vi "Host Approach RetractionA1copy-Aidan.vi"() -> ()   [LabVIEW 2012]
uses:
  <vilib>/Utility/file.llb/Write To Spreadsheet File (I64).vi
  <vilib>/FPGAPlugInAG/PCI-7831R/niLvFpga_Open_PCI-7831R.vi
  <vilib>/rvi/interface/common/dynamic/niFpgaDynamicAddResources.vi
  <vilib>/FPGAPlugInAG/Dynamic/niLvFpga_Run_Dynamic.vi
  <vilib>/Utility/error.llb/Error Cluster From Error Code.vi
  <vilib>/rvi/errors/niLvFpgaAdjustHostInterfaceError.vi
  <vilib>/FPGAPlugInAG/Dynamic/niLvFpga_Close_Dynamic.vi
  <vilib>/rvi/interface/nirviOpenFPGA/nirviOpenFPGA.xnode
  SB130-XPS/Documents/FPGA-project-apporach-retraction/FPGA Bitfiles/Apporach-Retract_FPGATarget2_FPGATargetApproa_sPWXUlF8ZuM.lvbitx
  Downloads/FPGA Target Approach RetractionA2copyAidanV2.vi
  <vilib>/rvi/interface/nirviMethod/nirviMethod.xnode
  <vilib>/rvi/interface/nirviReadWriteControl/nirviReadWriteControl.xnode
  <vilib>/rvi/interface/nirviCloseFPGA/nirviCloseFPGA.xnode
  <vilib>/rvi/interface/Simulation/niFpgaSimulationCallBeginRW.vi
  <vilib>/rvi/errors/niLvFpgaMergeErrorWithErrorCode.vi
  <vilib>/FPGAPlugInAG/Dynamic/niLvFpga_StartFifo_Dynamic.vi
  <vilib>/FPGAPlugInAG/Dynamic/niLvFpga_StopFifo_Dynamic.vi
  <vilib>/FPGAPlugInAG/Dynamic/niLvFpga_ReadFifo_Dynamic.vi
  NiFpgaLv.dll
panel:
  out "Acoustic Signal":u32[](graph)
  out "Acoustic Signal Data":i16[](array[numeric])
  in  "PANIC Retract\n\nApproach must be\n off before using":bool
  in  "File Name":string
  in  "Base Path":path
  in  "Colllect Data?":bool
  out "Counter Indicator Data":u16[](array[numeric])
  out "Total Error Data":u16[](array[numeric])
  out "Error Data":i16[](array[numeric])
  out "HV/10 Data":i16[](array[numeric])
  out "Tuning Fork \nSignal data":u16[](array[numeric])
  out "Counter Indicator":u32[](graph)
  out "Total Error":u16[](graph)
  out "Error":u16[](graph)
  out "Tuning Fork Signal":u16[](graph)
  out "HV/10":u16[](graph)
  out "Data 2":u64[](array[numeric])
  out "Data 1":u64[](array[numeric])
  in  "Intergral Constant":i32
  in  "Porportional Constant":i32
  in  "Feedback":bool
  in  "Approach Minimum":i32=20000
  in  "Approach Setpoint":i32=23000
  in  "Fast Approach Offset":i32=29000
  in  "TF in Air":i32=36000
  out "Fine A bits/us":dbl=5.463300000000001e-06
  out "Fine R bits/us":dbl=5.463300000000001e-06
  in  "Fine Approach (nm/s)":dbl=5.0
  in  "Fine Retraction (nm/s)":dbl=5.0
  out "Boolean 2":bool
  in  "DAQ Rate":i32=8000
  in  "Number of Elements":i32=100
  out "Fast A nm/s indicator":dbl=200.0
  out "Fast A bits/us":dbl=0.00021853200000000001
  out "Fast R nm/s indicator":dbl=200.0
  out "Fast R bits/us":dbl=0.00021853200000000001
  in  "Fast Approach (nm/s)":dbl=200.0
  in  "Fast Retraction (nm/s)":dbl=200.0
  in  "Automated Approach Start":bool
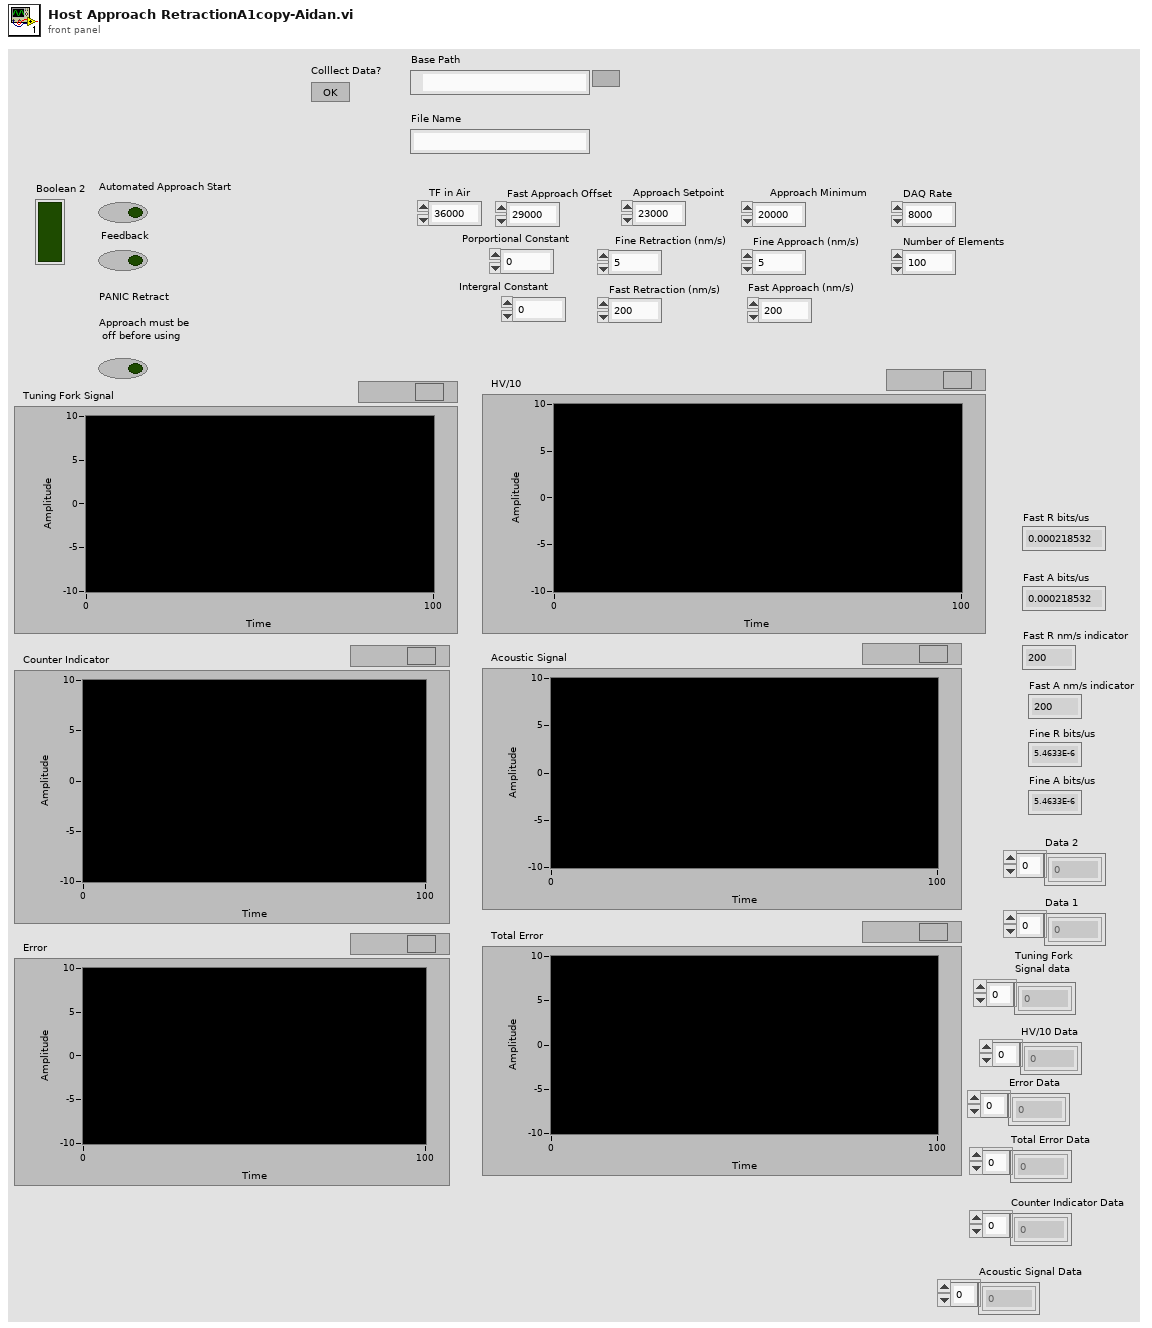
[diagram p1: front panel]
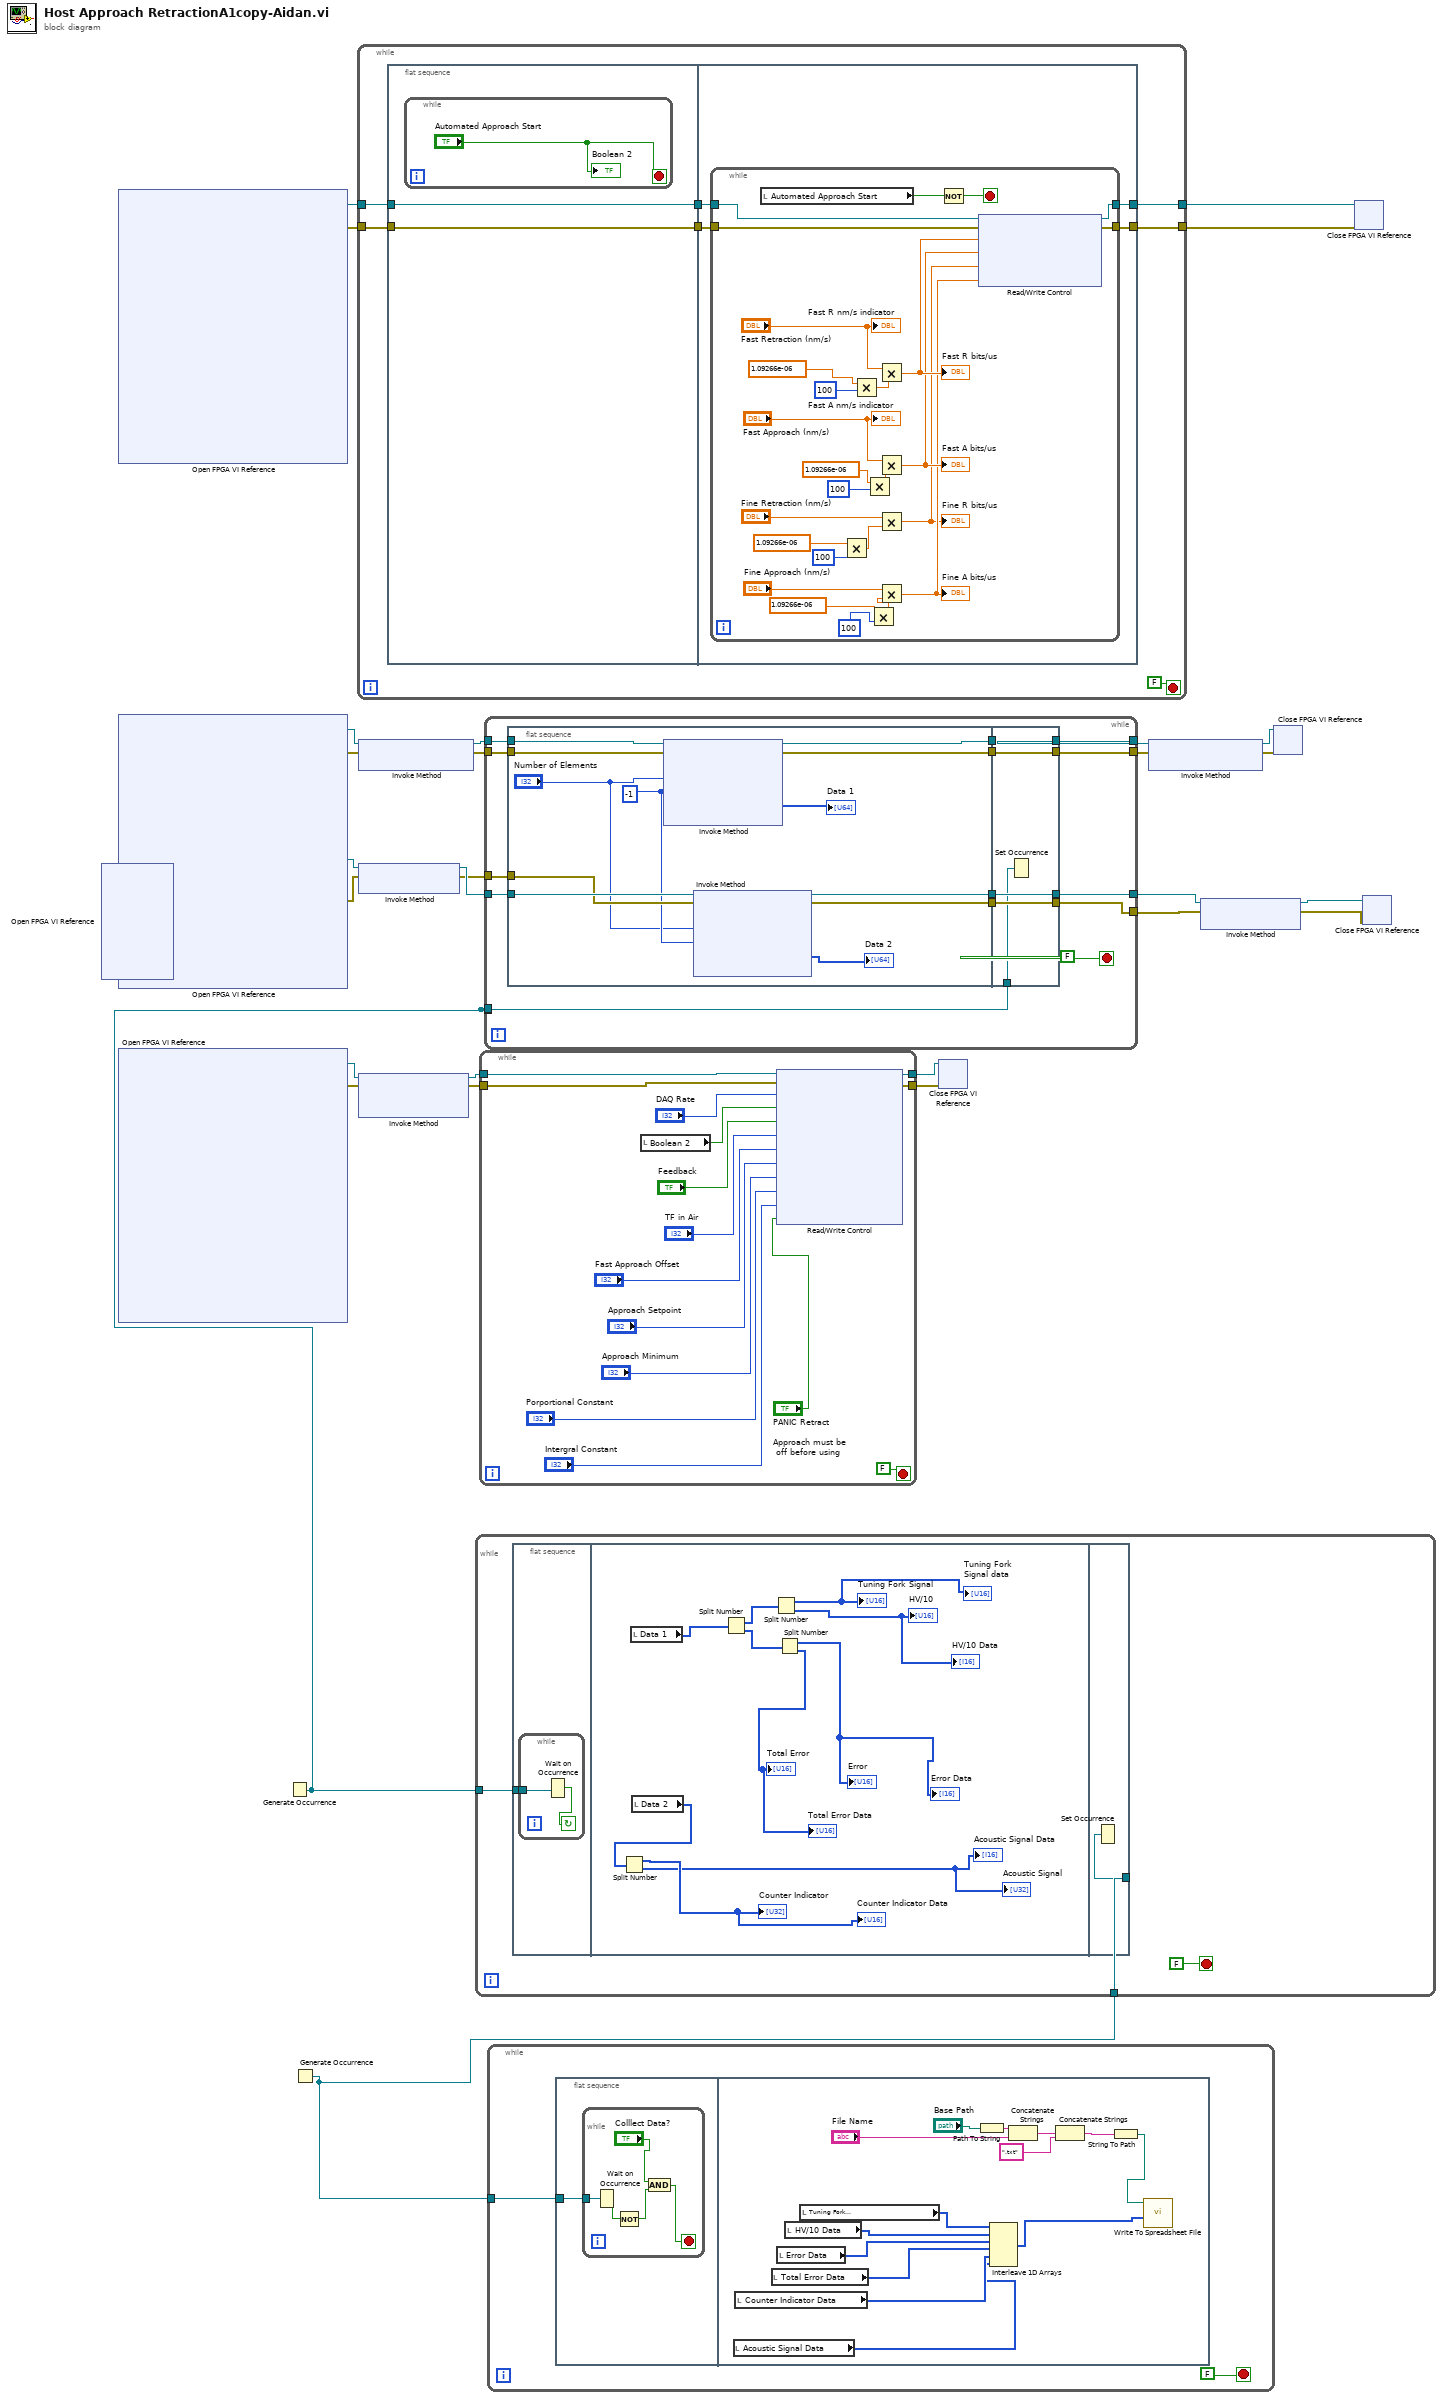
[diagram p0: block diagram]
diagram:
  n1 = xnode "Open FPGA VI Reference"() -> ("FPGA VI Reference Out"=w11:refnum<k20>, "error out"=w10:errorcluster)  [unwired: 2 in]
  n2 = xnode ("Open FPGA VI Reference")() -> ("FPGA VI Reference Out"=w23:refnum<k20>, "error out"=w22:errorcluster)  [unwired: 2 in]
  n3 = xnode "Open FPGA VI Reference"() -> ("FPGA VI Reference Out"=w9:refnum<k20>, "error out"=w19:errorcluster)  [unwired: 2 in]
  n4 = xnode "Open FPGA VI Reference"() -> ("FPGA VI Reference Out"=w24:refnum<k20>, "error out"=w12:errorcluster)  [unwired: 2 in]
  n5 = Generate Occurrence() -> (w2:refnum<k4>)
  n6 = Generate Occurrence() -> (w1:refnum<k4>)
  n7 = while {
    tunnel: w23 -> [w34]
    tunnel: w22 -> [w33]
    tunnel: [w30] -> w21
    tunnel: [w29] -> w20
    stop <- FALSE stop-if-true
    n8 = flat-sequence {
      tunnel: w34 -> [w37]
      tunnel: w33 -> [w36]
      tunnel: [w37] -> w32
      tunnel: [w36] -> w31
      tunnel: w32 -> [w42]
      tunnel: w31 -> [w41]
      tunnel: [w40] -> w30
      tunnel: [w39] -> w29
      frame #0 {
        n9 = while {
          stop <- "Automated Approach Start" stop-if-true
          "Boolean 2" <- "Automated Approach Start"
        }
      }
      frame #1 {
        n10 = while {
          tunnel: w42 -> [w62]
          tunnel: w41 -> [w61]
          tunnel: [w64] -> w40
          tunnel: [w63] -> w39
          stop <- w68 stop-if-true
          n11 = local read "Automated Approach Start"() -> (w67:bool)
          n12 = Multiply(x=1.09266e-06, y=100) -> (x*y=w47:dbl)
          n13 = Multiply(x=1.09266e-06, y=100) -> (x*y=w53:dbl)
          n14 = Multiply(x=1.09266e-06, y=100) -> (x*y=w50:dbl)
          n15 = Multiply(x=1.09266e-06, y=100) -> (x*y=w43:dbl)
          n16 = Multiply(x="Fast Retraction (nm/s)", y=w53) -> (x*y=w60:dbl)
          "Fast R bits/us" <- w60
          n17 = Multiply(x="Fast Approach (nm/s)", y=w50) -> (x*y=w59:dbl)
          "Fast A bits/us" <- w59
          n18 = Multiply(x="Fine Retraction (nm/s)", y=w47) -> (x*y=w55:dbl)
          "Fine R bits/us" <- w55
          n19 = Multiply(x="Fine Approach (nm/s)", y=w43) -> (x*y=w56:dbl)
          "Fine A bits/us" <- w56
          n20 = Not(x=w67) -> (.not. x?=w68:bool)
          n21 = xnode "Read/Write Control"("FPGA VI Reference In"=w62, "error in"=w61, "Fast Retraction Speed"=w60, "Fast Approach Speed"=w59, "Fine Retraction Speed"=w55, "Fine Approach Speed"=w56) -> ("FPGA VI Reference Out"=w64:refnum<k20>, "error out"=w63:errorcluster)
          "Fast R nm/s indicator" <- "Fast Retraction (nm/s)"
          "Fast A nm/s indicator" <- "Fast Approach (nm/s)"
        }
      }
    }
  }
  n22 = xnode "Invoke Method"("FPGA VI Reference In"=w9, "error in"=w19) -> ("FPGA VI Reference Out"=w18:refnum<k20>, "error out"=w17:errorcluster)
  n23 = xnode "Invoke Method"("FPGA VI Reference In"=w11, "error in"=w10) -> ("FPGA VI Reference Out"=w8:refnum<k20>, "error out"=w7:errorcluster)
  n24 = xnode "Invoke Method"("FPGA VI Reference In"=w24, "error in"=w12) -> ("FPGA VI Reference Out"=w26:refnum<k20>, "error out"=w25:errorcluster)  [unwired: 1 in]
  n25 = while {
    tunnel: w2 -> [w70]
    tunnel: w1 -> [w69]
    stop <- FALSE stop-if-true
    n26 = flat-sequence {
      tunnel: w70 -> [w72]
      tunnel: w69 -> [w85]
      frame #0 {
        n27 = while {
          tunnel: w72 -> [w74]
          stop <- w73 continue-if-true
          n28 = Wait on Occurrence(2:w74) -> (0:w73:bool)  [unwired: 2 in]
        }
      }
      frame #1 {
        n29 = local read "Data 1"() -> (w84:u64[])
        n30 = local read "Data 2"() -> (w77:u64[])
        n31 = Split Number(x=w77) -> (hi(x)=→"Counter Indicator" →"Counter Indicator Data":u32[], lo(x)=→"Acoustic Signal Data" →"Acoustic Signal":u32[])
        n32 = Split Number(x=w84) -> (hi(x)=w83:u32[], lo(x)=w82:u32[])
        n33 = Split Number(x=w83) -> (hi(x)=→"Tuning Fork Signal" →"Tuning Fork \nSignal data":u16[], lo(x)=→"HV/10" →"HV/10 Data":u16[])
        n34 = Split Number(x=w82) -> (hi(x)=→"Error" →"Error Data":u16[], lo(x)=→"Total Error" →"Total Error Data":u16[])
      }
      frame #2 {
        n35 = Set Occurrence(w85) -> ()
      }
    }
  }
  n36 = while {
    tunnel: w26 -> [w99]
    tunnel: w25 -> [w98]
    tunnel: [w97] -> w28
    tunnel: [w96] -> w27
    stop <- FALSE stop-if-true
    n37 = local read "Boolean 2"() -> (w94:bool)
    n38 = xnode "Read/Write Control"("FPGA VI Reference In"=w99, "error in"=w98, "Data Acquisition Rate"="DAQ Rate", "Approach"=w94, "Feedback?"="Feedback", "TF in Air"="TF in Air", "Fast Approach Offset"="Fast Approach Offset", "Approach Setpoint"="Approach Setpoint", "Approach Minimum"="Approach Minimum", "Porportional Constant"="Porportional Constant", "Integral Constant"="Intergral Constant", "PANIC Retract"="PANIC Retract\n\nApproach must be\n off before using") -> ("FPGA VI Reference Out"=w97:refnum<k20>, "error out"=w96:errorcluster)
  }
  n39 = while {
    tunnel: w18 -> [w114]
    tunnel: w17 -> [w113]
    tunnel: [w112] -> w16
    tunnel: [w111] -> w15
    tunnel: w8 -> [w109]
    tunnel: w7 -> [w108]
    tunnel: [w107] -> w6
    tunnel: [w106] -> w5
    tunnel: w2 -> [_]
    tunnel: w2 -> [w101]
    stop <- FALSE stop-if-true
    n40 = flat-sequence {
      tunnel: w114 -> [w126]
      tunnel: w113 -> [w125]
      tunnel: w109 -> [w122]
      tunnel: w108 -> [w121]
      tunnel: [w124] -> w105
      tunnel: [w123] -> w104
      tunnel: [w118] -> w103
      tunnel: [w117] -> w102
      tunnel: [w128] -> w106
      tunnel: [w129] -> w107
      tunnel: [w130] -> w111
      tunnel: [w131] -> w112
      tunnel: w105 -> [w131]
      tunnel: w104 -> [w130]
      tunnel: w103 -> [w129]
      tunnel: w102 -> [w128]
      tunnel: w101 -> [w127]
      frame #0 {
        w120 = -1
        n41 = xnode "Invoke Method"("FPGA VI Reference In"=w126, "error in"=w125, "Number of Elements"="Number of Elements", "Timeout (ms)"=w120) -> ("FPGA VI Reference Out"=w124:refnum<k20>, "error out"=w123:errorcluster, "Data"=→"Data 1":i64[])  [unwired: 1 out]
        n42 = xnode "Invoke Method"("FPGA VI Reference In"=w122, "error in"=w121, "Number of Elements"="Number of Elements", "Timeout (ms)"=w120) -> ("FPGA VI Reference Out"=w118:refnum<k20>, "error out"=w117:errorcluster, "Data"=→"Data 2":i16[])  [unwired: 1 out]
      }
      frame #1 {
        n43 = Set Occurrence(w127) -> ()
      }
    }
  }
  n44 = while {
    tunnel: w1 -> [w132]
    stop <- FALSE stop-if-true
    n45 = flat-sequence {
      tunnel: w132 -> [w134]
      frame #0 {
        n46 = while {
          tunnel: w134 -> [w135]
          stop <- w137 stop-if-true
          n47 = Wait on Occurrence(2:w135) -> (0:w136:bool)  [unwired: 2 in]
          n48 = Not(x=w136) -> (.not. x?=w138:bool)
          n49 = And(x="Colllect Data?", y=w138) -> (x .and. y?=w137:bool)
        }
      }
      frame #1 {
        n50 = local read "Acoustic Signal Data"() -> (w140:i16[])
        n51 = local read "Counter Indicator Data"() -> (w148:u16[])
        n52 = local read "Total Error Data"() -> (w152:u16[])
        n53 = local read "Error Data"() -> (w149:i16[])
        n54 = local read "HV/10 Data"() -> (w150:i16[])
        n55 = local read "Tuning Fork \nSignal data"() -> (w151:u16[])
        n56 = Path To String(path="Base Path") -> (string=w146:string)
        n57 = Interleave 1D Arrays(w151, w150, w149, w152, w148, w140) -> (w153:u16[])
        n58 = Concatenate Strings(w146, "File Name") -> (w144:string)
        n59 = Concatenate Strings(w144, ".txt") -> (w142:string)
        n60 = String To Path(string=w142) -> (path=w141:path)
        n61 = call-poly <vilib>:"Write To Spreadsheet File.vi"("1D data"=w153, "file path (dialog if empty)"=w141) -> ()  [unwired: 6 in, 1 out]
      }
    }
  }
  n62 = xnode "Close FPGA VI Reference"("FPGA VI Reference In"=w28, "error in"=w27) -> ()  [unwired: 1 out]
  n63 = xnode "Invoke Method"("FPGA VI Reference In"=w16, "error in"=w15) -> ("FPGA VI Reference Out"=w14:refnum<k20>, "error out"=w13:errorcluster)
  n64 = xnode "Invoke Method"("FPGA VI Reference In"=w6, "error in"=w5) -> ("FPGA VI Reference Out"=w4:refnum<k20>, "error out"=w3:errorcluster)
  n65 = xnode "Close FPGA VI Reference"("FPGA VI Reference In"=w14, "error in"=w13) -> ()  [unwired: 1 out]
  n66 = xnode "Close FPGA VI Reference"("FPGA VI Reference In"=w21, "error in"=w20) -> ()  [unwired: 1 out]
  n67 = xnode "Close FPGA VI Reference"("FPGA VI Reference In"=w4, "error in"=w3) -> ()  [unwired: 1 out]
